vi "test_generic.vi"() -> ()   [LabVIEW 2010, in "GenericImagingMode.lvclass"]
uses:
  GenericImagingMode.lvclass
  main/labview_source/type_definitions/enumerations/run_mode_enum.ctl
  main/labview_source/type_definitions/clusters/controls_refs.ctl
  common/classes/ErrorController/ErrorController/ErrorController.lvclass
  trigger_enum.ctl
  common/classes/ErrorController/ErrorController/class_data.vi
  common/classes/GenericComponent/GenericComponent/GenericComponent.lvclass
panel:
  out "error handler loaded?":bool
  in  "run mode":T1=enum."single sweep mode"
  in  "create and send":bool
  in  "start button":bool
  in  "proceed button":bool
  in  "stop":bool
  # "Test VI for ImagingMode components"
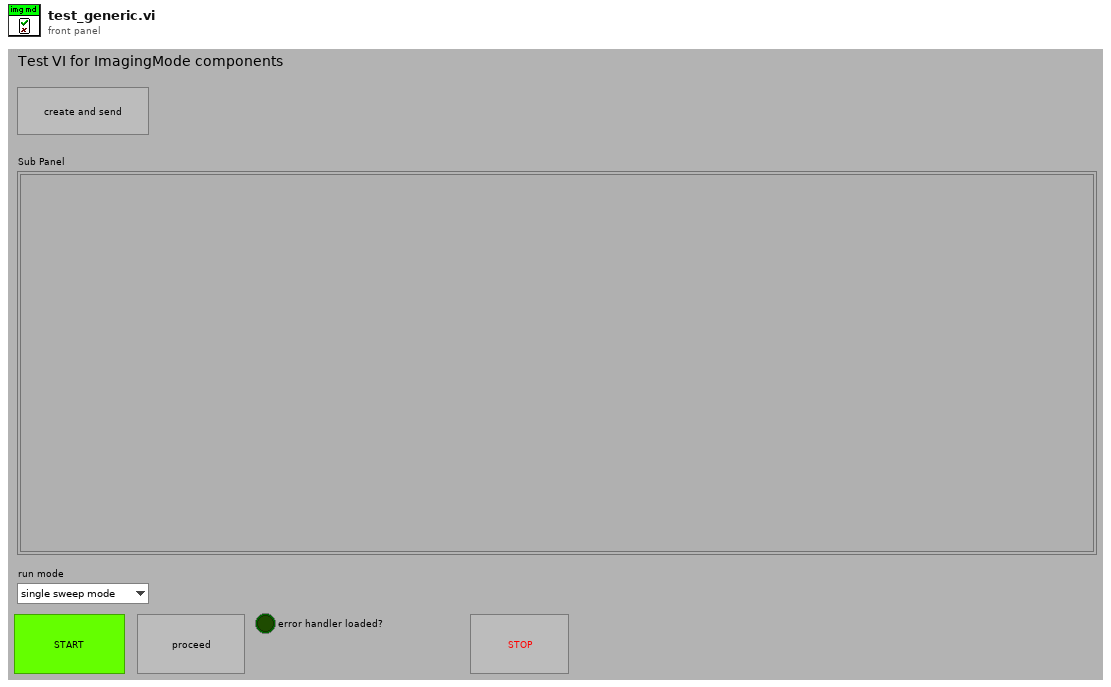
[diagram p1: front panel]
types:
  T1 = typedef "run_mode_enum.ctl" = enum16{"focus mode", "single sweep mode", "experiment mode"}
  T2 = typedef "controls_refs.ctl" = cluster{"scan start button":refnum<vi>, "tabs":cluster{"main":refnum<vi>, "settings":refnum<vi>}, "subpanels":cluster{"imagingMode":refnum<vi>, "scanHead":refnum<vi>, "display":refnum<vi>, "experimentController":refnum<vi>, "instrument":refnum<vi>, "stage":refnum<vi>, "stimulator":refnum<vi>, "dataCollection":refnum<vi>, "analyser":refnum<vi>, "daq":refnum<vi>, "imageAssembler":refnum<vi>}, "drop-downs":cluster{"run mode":refnum<vi>, "imagingMode":refnum<vi>, "experimentalController":refnum<vi>, "objective":refnum<vi>}, "status lights":cluster{"experimentController":refnum<vi>, "imagingMode":refnum<vi>, "scanHead":refnum<vi>, "daq":refnum<vi>, "imageAssembler":refnum<vi>, "dataCollection":refnum<vi>, "display":refnum<vi>, "analyser":refnum<vi>, "stage":refnum<vi>, "stimulator":refnum<vi>, "instrument":refnum<vi>}, "message":refnum<vi>, "stimulator enabled?":refnum<vi>, "saving":cluster{"data folder path":refnum<vi>, "file base name":refnum<vi>, "notebook":refnum<vi>}, "progress bar":refnum<vi>, "update icon":refnum<vi>, "title":refnum<vi>, "main vi":refnum<vi>, "user":refnum<vi>, "exit_button":refnum<vi>, "CPU usage %":refnum<vi>}
  T3 = typedef "GenericImagingMode.lvclass/trigger_enum.ctl" = enum16{"NULL", "start", "stop", "proceed"}
  T4 = typedef "XComponentSpecification.xctl/data.ctl" = cluster{"class path":string, "configuration":string, "label":string, "settings name":string}
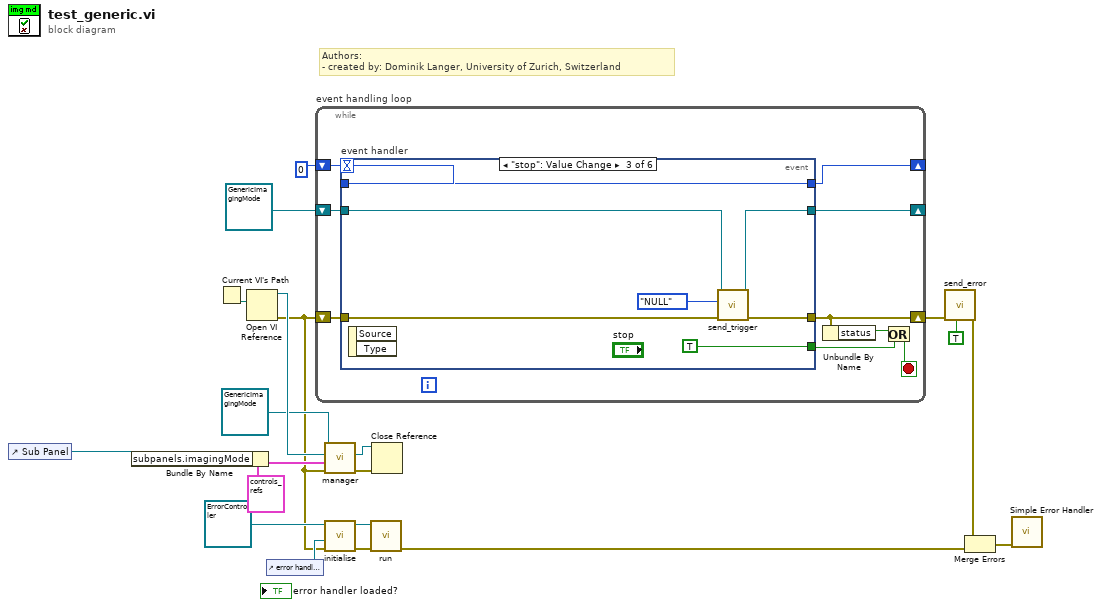
[diagram p0: block diagram]
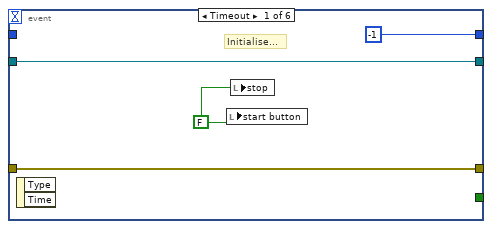
[diagram p2: hidden frame]
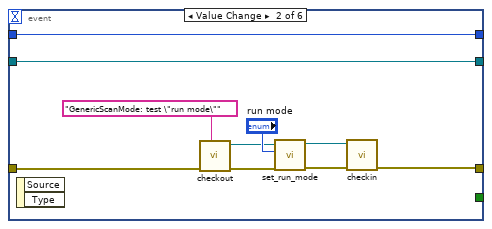
[diagram p3: hidden frame]
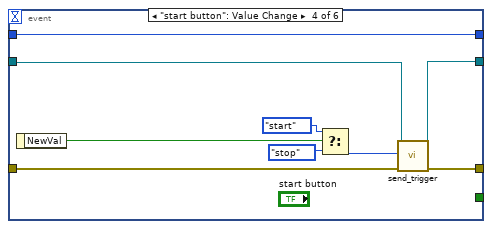
[diagram p4: hidden frame]
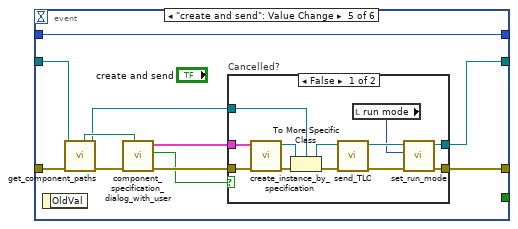
[diagram p5: hidden frame]
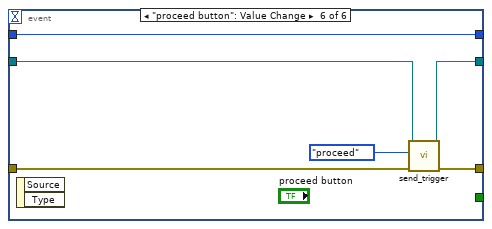
[diagram p7: hidden frame]
diagram:
  # "Authors: \n- created by: Dominik Langer, University of Zurich, Switzerland"
  n1 = control-ref of="Sub Panel"() -> (w18:refnum<vi>)
  n2 = Bundle By Name(cluster=T2 {"scan start button"=refnum, "tabs"={"main"=refnum, "settings"=refnum}, "subpanels"={"imagingMode"=refnum, "scanHead"=refnum, "display"=refnum, "experimentController"=refnum, "instrument"=refnum, "stage"=refnum, "stimulator"=refnum, "dataCollection"=refnum, "analyser"=refnum, "daq"=refnum, "imageAssembler"=refnum}, "drop-downs"={"run mode"=refnum, "imagingMode"=refnum, "experimentalController"=refnum, "objective"=refnum}, "status lights"={"experimentController"=refnum, "imagingMode"=refnum, "scanHead"=refnum, "daq"=refnum, "imageAssembler"=refnum, "dataCollection"=refnum, "display"=refnum, "analyser"=refnum, "stage"=refnum, "stimulator"=refnum, "instrument"=refnum}, "message"=refnum, "stimulator enabled?"=refnum, "saving"={"data folder path"=refnum, "file base name"=refnum, "notebook"=refnum}, "progress bar"=refnum, "update icon"=refnum, "title"=refnum, "main vi"=refnum, "user"=refnum, "exit_button"=refnum, "CPU usage %"=refnum} ("control references"), "subpanels.imagingMode"=w18) -> (w14:T2)
  n3 = Current VI's Path() -> (path=w17:path)
  n4 = Open VI Reference(vi path=w17) -> (vi reference=w13:refnum<vi>, error out=w6:errorcluster)  [unwired: 1 in, 4 out]
  n5 = control-ref of="error handler loaded?"() -> (w10:refnum<vi>)
  n6 = while "event handling loop" {
    shift-right: [w24] -> w4
    shift-left: w6 -> [w29]
    shift-right: [w27] -> _
    shift-left: 0 -> [w28]
    shift-right: [w25] -> _
    shift-left: refnum<class "GenericImagingMode.lvclass"> refnum ("GenericImagingMode.lvclass") -> [w26]
    stop <- w21 stop-if-true
    n7 = event "event handler" shown="[2] \"stop\": Value Change" {
      selector: _ -> [_ _ _ _ _ _]
      dyn-events: _ -> [_ _ _ _ _ _]
      timeout: w28 -> [_ _ _ _ _ _]
      tunnel: w29 -> [w30 w41 w48 w54 w65 w89]
      tunnel: [_ _ TRUE _ _ _] -> w22
      tunnel: [w30 w38 w47 w53 w68 w88] -> w24
      tunnel: [-1 w43 w49 w59 w70 w90] -> w27
      tunnel: w28 -> [_ w43 w49 w59 w70 w90]
      tunnel: [w31 w42 w45 w51 w69 w85] -> w25
      tunnel: w26 -> [w31 w42 w46 w52 w63 w86]
      event Timeout {
        w32 = FALSE
        # "Initialise..."
        n8 = event-data() -> ()  [unwired: 3 out]
        n9 = local write "start button"(w32) -> ()
        n10 = local write "stop"(w32) -> ()
      }
      event Value Change {
        n11 = event-data() -> ()  [unwired: 3 out]
        n12 = call "checkout.vi"("locked by?"="GenericScanMode: test \"run mode\"", "error in (no error)"=w41) -> ("error out"=w40:errorcluster, "GenericScanMode out"=w36:refnum<class "GenericImagingMode.lvclass">)  [unwired: 8 out]
        n13 = call-dynamic "set_run_mode.vi"("error in (no error)"=w40, "run mode"="run mode", "GenericPlugin in"=w36) -> ("error out"=w39:errorcluster, "GenericPlugin out"=w35:refnum<class "GenericImagingMode.lvclass">)  [unwired: 7 out]
        n14 = call-dynamic "checkin.vi"("error in (no error)"=w39, "GenericScanMode in"=w35) -> ("error out"=w38:errorcluster)  [unwired: 8 in, 1 out]
      }
      event "stop": Value Change {
        n15 = event-data() -> ()  [unwired: 3 out]
        n16 = call-dynamic "send_trigger.vi"("error in (no error)"=w48, "message"=trigger_enum."NULL", "GenericScanMode in"=w46) -> ("error out"=w47:errorcluster, "GenericScanMode out"=w45:refnum<class "GenericImagingMode.lvclass">)  [unwired: 7 out]
      }
      event "start button": Value Change {
        n17 = event-data() -> ("NewVal"=w58:bool)  [unwired: 1 out]
        n18 = Select(t=trigger_enum."start" ("message"), s=w58, f=trigger_enum."stop" ("message")) -> (s? t:f=w55:T3)
        n19 = call-dynamic "send_trigger.vi"("error in (no error)"=w54, "message"=w55, "GenericScanMode in"=w52) -> ("error out"=w53:errorcluster, "GenericScanMode out"=w51:refnum<class "GenericImagingMode.lvclass">)  [unwired: 7 out]
      }
      event "create and send": Value Change {
        n20 = event-data() -> ()  [unwired: 2 out]
        n21 = call-dynamic "get_component_paths.vi"("error in (no error)"=w65, "GenericComponent in"=w63) -> ("error out"=w67:errorcluster, "GenericComponent out"=w62:refnum<class "GenericImagingMode.lvclass">, "component type directory"=w66:path)  [unwired: 4 in, 3 out]
        n22 = call "component_specification_dialog_with_user.vi"("start path"=w66, "error in (no error)"=w67) -> ("error out"=w64:errorcluster, "cancelled?"=w61:bool, "component specification out"=w60:T4)  [unwired: 7 in]
        n23 = case "Cancelled?" shown="False" w61 {
          tunnel: [w81 w83] -> w69
          tunnel: [w79 w84] -> w68
          tunnel: w64 -> [w73 w84]
          tunnel: w62 -> [w72 w83]
          tunnel: w60 -> [w71 _]
          frame False {
            n24 = call "create_instance_by_specification.vi"("error in (no error)"=w73, "component specification"=w71) -> ("error out"=w77:errorcluster, "GenericPlugin out"=w74:refnum<class "GenericComponent.lvclass">)  [unwired: 7 in, 1 out]
            n25 = To More Specific Class(target class=w72, reference=w74, error in=w77) -> (specific class reference=w75:refnum<class "GenericImagingMode.lvclass">, error out=w76:errorcluster)
            n26 = call-dynamic "send_TLC.vi"("error in (no error)"=w76, "GenericToplevelComponent in"=w75) -> ("error out"=w80:errorcluster, "GenericToplevelComponent out"=w82:refnum<class "GenericImagingMode.lvclass">)  [unwired: 8 out]
            n27 = local read "run mode"() -> (w78:T1)
            n28 = call-dynamic "set_run_mode.vi"("error in (no error)"=w80, "run mode"=w78, "GenericPlugin in"=w82) -> ("error out"=w79:errorcluster, "GenericPlugin out"=w81:refnum<class "GenericImagingMode.lvclass">)  [unwired: 7 out]
          }
          frame True {
          }
        }
      }
      event "proceed button": Value Change {
        n29 = event-data() -> ()  [unwired: 3 out]
        n30 = call-dynamic "send_trigger.vi"("error in (no error)"=w89, "message"=trigger_enum."proceed", "GenericScanMode in"=w86) -> ("error out"=w88:errorcluster, "GenericScanMode out"=w85:refnum<class "GenericImagingMode.lvclass">)  [unwired: 7 out]
      }
    }
    n31 = Unbundle By Name(w24) -> ("status"=w23:bool)
    n32 = Or(x=w23, y=w22) -> (x .or. y?=w21:bool)
  }
  n33 = call-dynamic "manager.vi"("error in (no error)"=w6, "control references"=w14, "top-level VI ref in"=w13, "GenericToplevelComponent in"=refnum<class "GenericImagingMode.lvclass"> refnum ("GenericImagingMode.lvclass")) -> ("error out"=w15:errorcluster, "top-level VI ref out"=w12:refnum<vi>)  [unwired: 5 in, 1 out]
  n34 = call-dynamic "initialise.vi"("error in (no error)"=w6, "error boolean"=w10, "ErrorController in"=refnum<class "ErrorController.lvclass"> refnum) -> ("error out"=w9:errorcluster, "ErrorController out"=w8:refnum<class "ErrorController.lvclass">)  [unwired: 7 in]
  n35 = call "run.vi"("error in (no error)"=w9, "ErrorController in"=w8) -> ("error out"=w2:errorcluster)  [unwired: 8 in, 1 out]
  n36 = Close Reference(reference=w12, error in (no error)=w15) -> ()  [unwired: 1 out]
  n37 = call "send_error.vi"("last error? (F)"=TRUE, "error in (no error)"=w4) -> ("error out"=w3:errorcluster)  [unwired: 9 in]
  n38 = Merge Errors(w3, w2) -> (w5:errorcluster)
  n39 = call <vilib>:"Simple Error Handler.vi"("error in (no error)"=w5) -> ()  [unwired: 4 in, 5 out]
